vi "Own_Code_BB.vi"() -> ()   [LabVIEW 2012]
uses:
  SubVIs/LVPresent_Globals.vi
panel:
  in  "Tab Control":enum32{"Page 1", "Page 2"}(tab)
  in  "Circuit":bool
  in  "Open":bool
  in  "Solution":bool
  in  "Back":bool
  # "Let's try some coding!\n\nClick the \"Open\" button below to start a blank VI. Click the image to the right (the \"Beaglebutton\") to see how to construct the circuit. This will be similar to the examples you just did, but using an LED on a breadboard instead of on the BeagleBone. Pin 11 is pin 4 in LabVIEW."
  # "Let's start by simply turning the LED on. Then have it turn off after a certain amount of time (like the second example you just did). Finally, use a For Loop to have it blink 5 times. Check out the help if you have any issues!"
  # "Remember to have the program wait again after the light turns off when you are making it blink."
  # "330½ Resistor"
  # "GND Pin"
  # "LED"
  # "Pin 11"
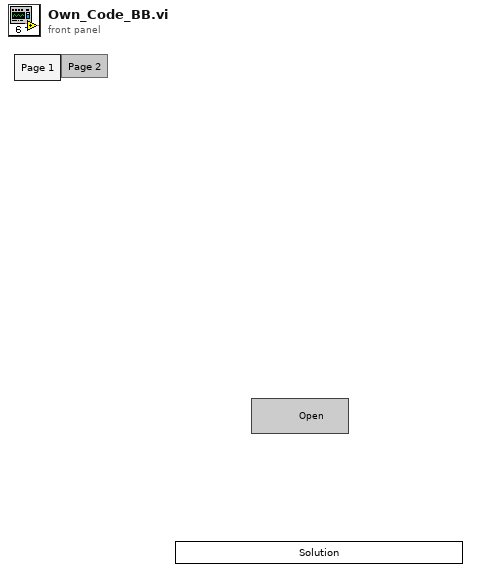
[diagram p1: front panel]
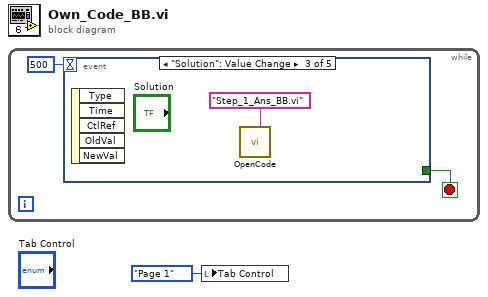
[diagram p0: block diagram]
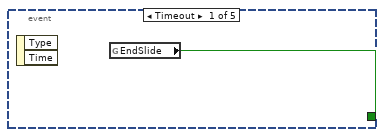
[diagram p2: hidden frame]
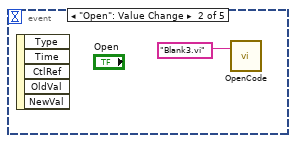
[diagram p3: hidden frame]
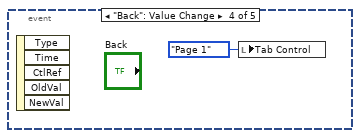
[diagram p4: hidden frame]
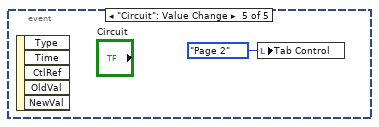
[diagram p5: hidden frame]
diagram:
  n1 = while {
    stop <- w3 stop-if-true
    n2 = event shown="[2] \"Solution\": Value Change" {
      selector: _ -> [_ _ _ _ _]
      dyn-events: _ -> [_ _ _ _ _]
      timeout: 500 -> [_ _ _ _ _]
      tunnel: [w4 _ _ _ _] -> w3
      event Timeout {
        n3 = event-data() -> ()  [unwired: 1 in, 2 out]
        n4 = global read "LVPresent_Globals.vi" "EndSlide"() -> (w4:bool)
      }
      event "Open": Value Change {
        n5 = event-data() -> ()  [unwired: 1 in, 5 out]
        n6 = call "OpenCode.vi"("Code name"="Blank3.vi") -> ()  [unwired: 3 in]
      }
      event "Solution": Value Change {
        n7 = event-data() -> ()  [unwired: 1 in, 5 out]
        n8 = call "OpenCode.vi"("Code name"="Step_1_Ans_BB.vi") -> ()  [unwired: 3 in]
      }
      event "Back": Value Change {
        n9 = event-data() -> ()  [unwired: 1 in, 5 out]
        n10 = local write "Tab Control"(enum32{"Page 1", "Page 2"}."Page 1" ("Tab Control")) -> ()
      }
      event "Circuit": Value Change {
        n11 = event-data() -> ()  [unwired: 1 in, 5 out]
        n12 = local write "Tab Control"(enum32{"Page 1", "Page 2"}."Page 2" ("Tab Control")) -> ()
      }
    }
  }
  n13 = local write "Tab Control"(enum32{"Page 1", "Page 2"}."Page 1" ("Tab Control")) -> ()
